vi "Open VIRef to Compile.vi"(8 "error in (no error)":errorcluster, 10 "milliseconds to wait":u32, 11 "dup path":path) -> (0 "error out":errorcluster)   [LabVIEW 2017]
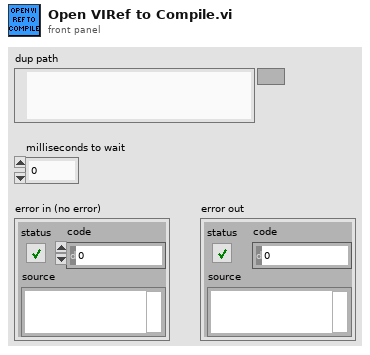
[diagram p1: front panel]
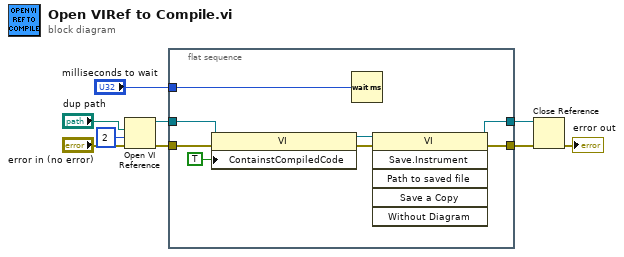
[diagram p0: block diagram]
diagram:
  n1 = Open VI Reference(vi path="dup path", options=2, error in (no error)="error in (no error)") -> (vi reference=w5:refnum<vi>, error out=w1:errorcluster)  [unwired: 3 in]
  n2 = flat-sequence {
    tunnel: w1 -> [w17]
    tunnel: [w16] -> w2
    tunnel: [w15] -> w4
    tunnel: w5 -> [w13]
    tunnel: "milliseconds to wait" -> [w10]
    frame #0 {
      n3 = property class="VI"(reference=w13, error in=w17, "ContainstCompiledCode"=TRUE ("Contains Compiled Code")) -> (reference out=w12:refnum<vi>, error out=w14:errorcluster)
      n4 = Wait (ms)(milliseconds to wait=w10) -> ()  [unwired: 1 out]
      n5 = invoke class="VI" method="Save.Instrument"(reference=w12, error in=w14) -> (reference out=w15:refnum<vi>, error out=w16:errorcluster)  [unwired: 4 in, 4 out]
    }
  }
  n6 = Close Reference(reference=w4, error in (no error)=w2) -> (error out=→"error out":errorcluster)
